vi "ShoulderGetPositionDemand.vi"() -> (7 "ShoulderPosDmdDeg":dbl)   [LabVIEW 2023]
uses:
  ShoulderGlobal.vi
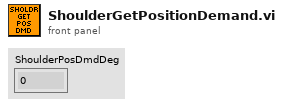
[diagram p1: front panel]
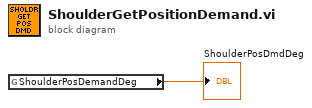
[diagram p0: block diagram]
diagram:
  n1 = global read "ShoulderGlobal.vi" "ShoulderPosDemandDeg"() -> (→"ShoulderPosDmdDeg":dbl)
